vi "load class.vi"(8 "error in":errorcluster, 9 "available class paths":path[](array[path]), 10 "available class names":string[](array[string]), 11 "Class Name":string) -> (0 "error out":errorcluster, 3 "Object Out":refnum<class>)   [LabVIEW 2013, in "class discovery singleton.lvlib"]
doc: "Attempts to load a class, by name, either from memory or from disk. First it tries the exact name in memory. Then it tries the filename on disk. Then it tries an approximate match of all VIs in memory."
uses:
  class discovery singleton.lvlib
  <vilib>/NI/Tag Bus Module Framework/root configuration/TBM configuration.lvclass
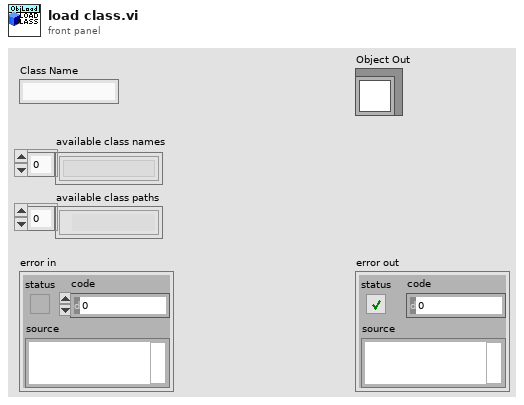
[diagram p1: front panel]
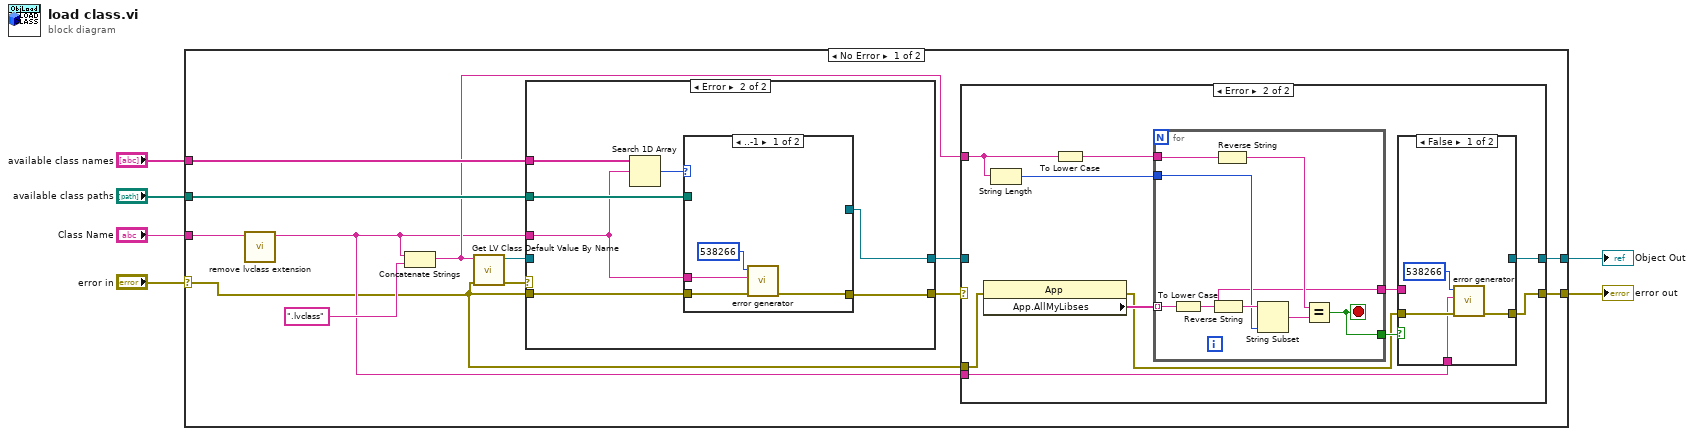
[diagram p0: block diagram]
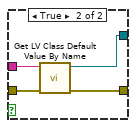
[diagram p3: hidden frame]
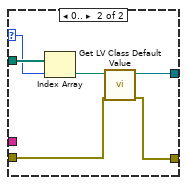
[diagram p5: hidden frame]
diagram:
  n1 = case shown="No Error" "error in" {
    selector: "error in" -> [w7 w68]
    tunnel: "Class Name" -> [w15 _]
    tunnel: [w13 _] -> w3
    tunnel: [w11 w68] -> w4
    tunnel: "available class paths" -> [w17 _]
    tunnel: "available class names" -> [w16 _]
    frame No Error {
      n2 = call "remove lvclass extension.vi"("class name in"=w15) -> ("class name out"=w8:string)  [unwired: 10 in]
      n3 = Concatenate Strings(w8, ".lvclass" ("string")) -> (w9:string)
      n4 = call <vilib>:"Get LV Class Default Value By Name.vi"("error in (no error)"=w7, "class name"=w9) -> ("error out"=w19:errorcluster, "object"=w18:refnum<class>)  [unwired: 8 in]
      n5 = case shown="Error" w19 {
        selector: w19 -> [w50 _]
        tunnel: w18 -> [w49 _]
        tunnel: w8 -> [_ w51]
        tunnel: [w50 w56] -> w10
        tunnel: [w49 w57] -> w12
        tunnel: w17 -> [_ w53]
        tunnel: w16 -> [_ w55]
        tunnel: w7 -> [_ w52]
        frame No Error {
        }
        frame Error {
          n6 = Search 1D Array(1D array=w55, element=w51) -> (index of element=w54:i32)  [unwired: 1 in]
          n7 = case shown="..-1" w54 {
            selector: w54 -> [_ w63]
            tunnel: [w60 w67] -> w56
            tunnel: [_ w66] -> w57
            tunnel: w53 -> [_ w65]
            tunnel: w52 -> [w61 w62]
            tunnel: w51 -> [w58 _]
            frame ..-1 {
              n8 = call <vilib>:"error generator.vi"("error in"=w61, "append error message"=w58, "error code (0)"=538266) -> ("error out"=w60:errorcluster)  [unwired: 8 in]
            }
            frame 0.. {
              n9 = Index Array(array=w65, index=w63) -> (element=w64:path)
              n10 = call <vilib>:"Get LV Class Default Value.vi"("error in (no error)"=w62, "class path"=w64) -> ("error out"=w67:errorcluster, "object"=w66:refnum<class>)  [unwired: 8 in]
            }
          }
        }
      }
      n11 = case shown="Error" w10 {
        selector: w10 -> [w20 _]
        tunnel: [w21 w24] -> w13
        tunnel: w12 -> [w21 _]
        tunnel: [w20 w25] -> w11
        tunnel: w7 -> [_ w32]
        tunnel: w9 -> [_ w30]
        tunnel: w8 -> [_ w23]
        frame No Error {
        }
        frame Error {
          n12 = property class="App"(error in=w32) -> (error out=w26:errorcluster, "App.AllMyLibses"=w31:string[])  [unwired: 1 in, 1 out]
          n13 = String Length(string=w30) -> (length=w29:i32)
          n14 = To Lower Case(string=w30) -> (all lower case string=w22:string)
          n15 = for {
            tunnel: w31 -> [w43] mode=indexing
            tunnel: w22 -> [w48]
            tunnel: w29 -> [w46]
            tunnel: [w41] -> w28
            tunnel: [w42] -> w27
            stop <- w42 stop-if-true
            n16 = To Lower Case(string=w43) -> (all lower case string=w41:string)
            n17 = Reverse String(1:w41) -> (0:w47:string)
            n18 = Reverse String(1:w48) -> (0:w44:string)
            n19 = String Subset(string=w47, length (rest)=w46) -> (substring=w45:string)  [unwired: 1 in]
            n20 = Equal?(x=w44, y=w45) -> (x = y?=w42:bool)
          }
          n21 = case shown="False" w27 {
            tunnel: w28 -> [_ w40]
            tunnel: w26 -> [w34 w39]
            tunnel: [w35 w38] -> w25
            tunnel: [_ w37] -> w24
            tunnel: w23 -> [w33 _]
            frame False {
              n22 = call <vilib>:"error generator.vi"("error in"=w34, "append error message"=w33, "error code (0)"=538266) -> ("error out"=w35:errorcluster)  [unwired: 8 in]
            }
            frame True {
              n23 = call <vilib>:"Get LV Class Default Value By Name.vi"("error in (no error)"=w39, "class name"=w40) -> ("error out"=w38:errorcluster, "object"=w37:refnum<class>)  [unwired: 8 in]
            }
          }
        }
      }
    }
    frame Error {
    }
  }
  "error out" <- w4
  "Object Out" <- w3
